vi "Posiion rediction.vi"(7 "Nr of particles":dbl, 8 "Hover":bool, 9 "Current Position":T1, 10 "Roll":dbl, 11 "Pitch":dbl) -> (0 "Hover Out":bool, 2 "Roll Out":dbl, 3 "Pitch Out":dbl)   [LabVIEW 2014]
uses:
  Global.vi
panel:
  out "Boolean":bool
  in  "Enable Prediction":bool=TRUE
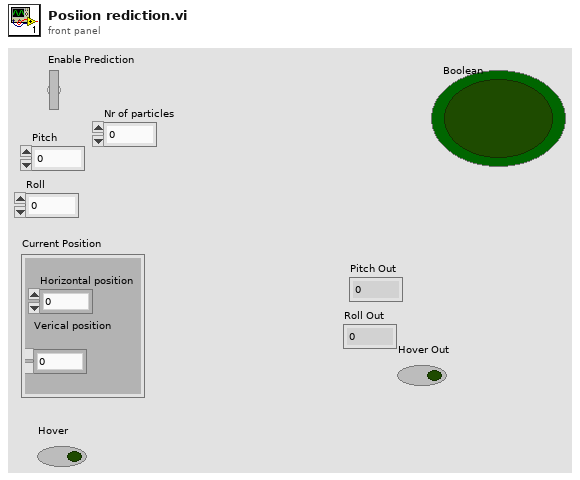
[diagram p1: front panel]
types:
  T1 = cluster{"Horizontal position":dbl, "Verical position\n":dbl}
  T2 = typedef "AR Drone.lvlib/NavData Demo.ctl" = cluster{"control state":enum32{"DEFAULT", "INIT", "LANDING", "FLYING", "HOVERING", "TEST", "TRANS_TAKEOFF", "TRANS_GOTOFIX", "TRANS_LANDING"}, "battery percentage":u32, "pitch (deg)":sgl, "roll (deg)":sgl, "yaw (deg)":sgl, "altitude (cm)":u32, "vx (cm/s)?":sgl, "vy (cm/s)?":sgl, "vz (cm/s)?":sgl, "detection cam type":u32}
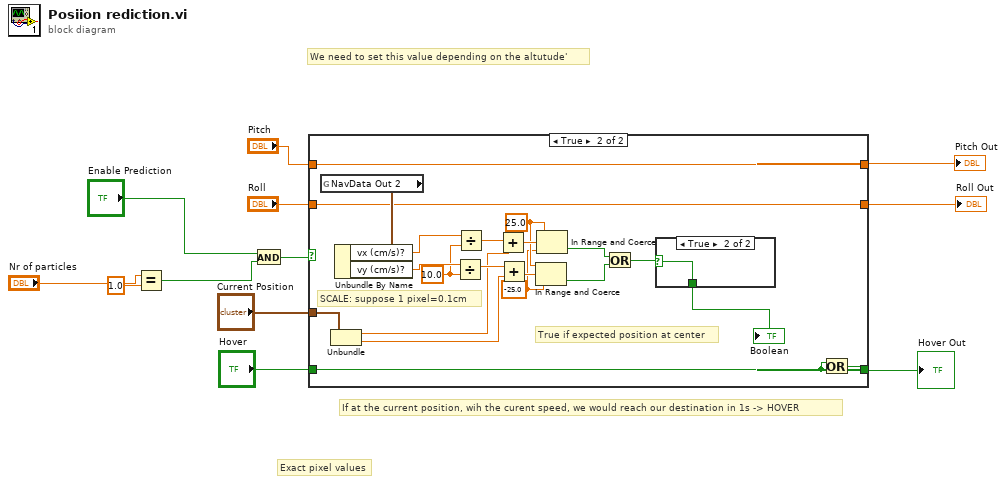
[diagram p0: block diagram]
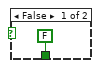
[diagram p3: hidden frame]
diagram:
  # "We need to set this value depending on the altutude'"
  # "Exact pixel values"
  # "If at the current position, wih the curent speed, we would reach our destination in 1s -> HOVER"
  n1 = Equal?(x="Nr of particles", y=1.0) -> (x = y?=w2:bool)
  n2 = And(x="Enable Prediction", y=w2) -> (x .and. y?=w1:bool)
  n3 = case shown="True" w1 {
    tunnel: "Pitch" -> [w15 w32]
    tunnel: "Roll" -> [w14 w33]
    tunnel: [w15 w32] -> w10
    tunnel: [w14 w33] -> w9
    tunnel: "Hover" -> [w13 w16]
    tunnel: [w13 w35] -> w7
    tunnel: "Current Position" -> [_ w34]
    frame False {
    }
    frame True {
      w19 = 25.0 ("upper limit")
      w18 = -25.0 ("lower limit")
      w29 = sgl 10.0 ("y")
      # "True if expected position at center"
      # "SCALE: suppose 1 pixel=0.1cm"
      n4 = global read "Global.vi" "NavData Out 2"() -> (w36:T2)
      n5 = Unbundle(w34) -> ("Horizontal position"=w26:dbl, "Verical position"=w25:dbl)
      n6 = Unbundle By Name(w36) -> ("vx (cm/s)?"=w31:sgl, "vy (cm/s)?"=w30:sgl)
      n7 = Divide(x=w30, y=w29) -> (x/y=w27:sgl)
      n8 = Divide(x=w31, y=w29) -> (x/y=w28:sgl)
      n9 = Add(x=w28, y=w26) -> (x+y=w21:dbl)
      n10 = Add(x=w27, y=w25) -> (x+y=w20:dbl)
      n11 = In Range and Coerce(upper limit=w19, x=w20, lower limit=w18) -> (In Range?=w23:bool)  [unwired: 1 out]
      n12 = In Range and Coerce(upper limit=w19, x=w21, lower limit=w18) -> (In Range?=w22:bool)  [unwired: 1 out]
      n13 = Or(x=w22, y=w23) -> (x .or. y?=w24:bool)
      n14 = case shown="True" w24 {
        selector: w24 -> [_ w38]
        tunnel: [FALSE w38] -> w17
        frame False {
        }
        frame True {
        }
      }
      "Boolean" <- w17
      n15 = Or(x=w16, y=w16) -> (x .or. y?=w35:bool)
    }
  }
  "Pitch Out" <- w10
  "Roll Out" <- w9
  "Hover Out" <- w7
